vi "DAQ_Read.vi"(3 "error in":errorcluster, 4 "Samples per Read":i32, 5 "task in":refnum<k21>) -> (0 "error out":errorcluster, 1 "Y array":dbl, 2 "X array":dbl)   [LabVIEW 2024]
uses:
  <vilib>/DAQmx/read.llb/DAQmx Read (Analog 2D DBL NChan NSamp).vi
  <vilib>/DAQmx/miscellaneous.llb/DAQmx Fill In Error Info.vi
panel:
  in  "array":dbl[](array[numeric])
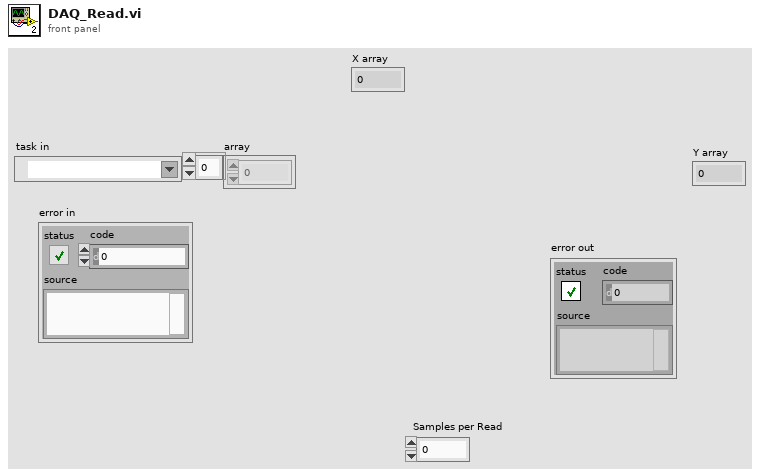
[diagram p1: front panel]
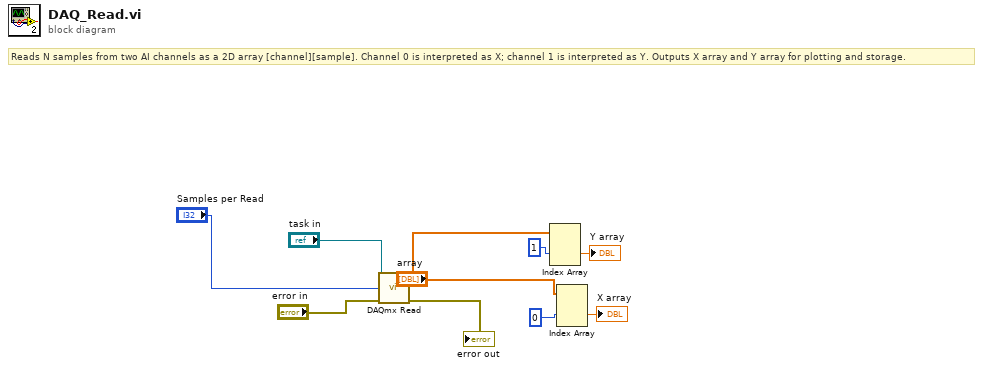
[diagram p0: block diagram]
diagram:
  # "Reads N samples from two AI channels as a 2D array [channel][sample]. Channel 0 is interpreted as X; channel 1 is interpreted as Y. Outputs X array and Y array for plotting and storage."
  n1 = call-poly <vilib>:"DAQmx Read.vi"("task/channels in"="task in", "number of samples per channel"="Samples per Read", "error in"="error in") -> ("error out"=→"error out":errorcluster)  [unwired: 10 in, 2 out]
  n2 = Index Array(array="array", index #2=1 ("index")) -> (element #2=→"Y array":dbl)  [unwired: 2 in, 2 out]
  n3 = Index Array(array="array", index #2=0 ("index (row)")) -> (element #2=→"X array":dbl)  [unwired: 2 in, 2 out]
